vi "motor run.vi"(8 "error in (no error)":errorcluster, 9 "reset":bool, 10 "speed":dbl, 11 "motor in":refnum<class "motor.lvclass">) -> (0 "error out":errorcluster, 3 "motor out":refnum<class "motor.lvclass">)   [LabVIEW 2019, in "my FPGA lib.lvlib" / "motor.lvclass"]
uses:
  motor.lvclass
  motor.lvclass/motor.ctl
  control/PID control.ctl
panel:
  out "motor encoder(degrees)":dbl
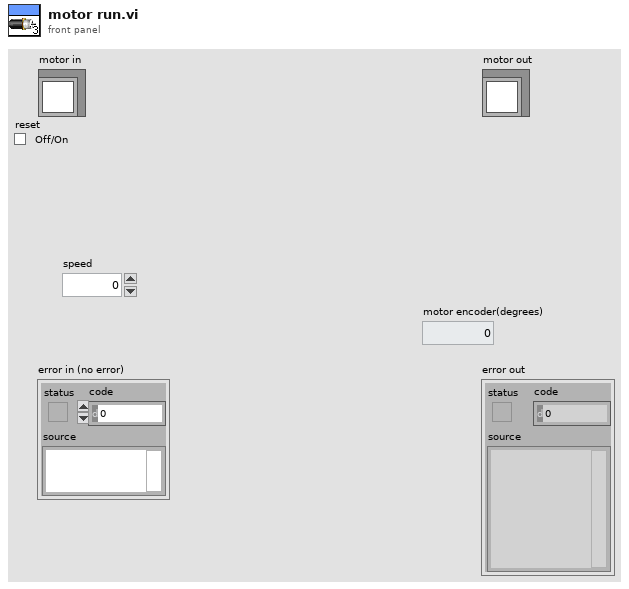
[diagram p1: front panel]
types:
  T1 = typedef "my FPGA lib.lvlib/motor.lvclass/PID control.ctl" = cluster{"setpoint":dbl, "processer":dbl, "last output":dbl}
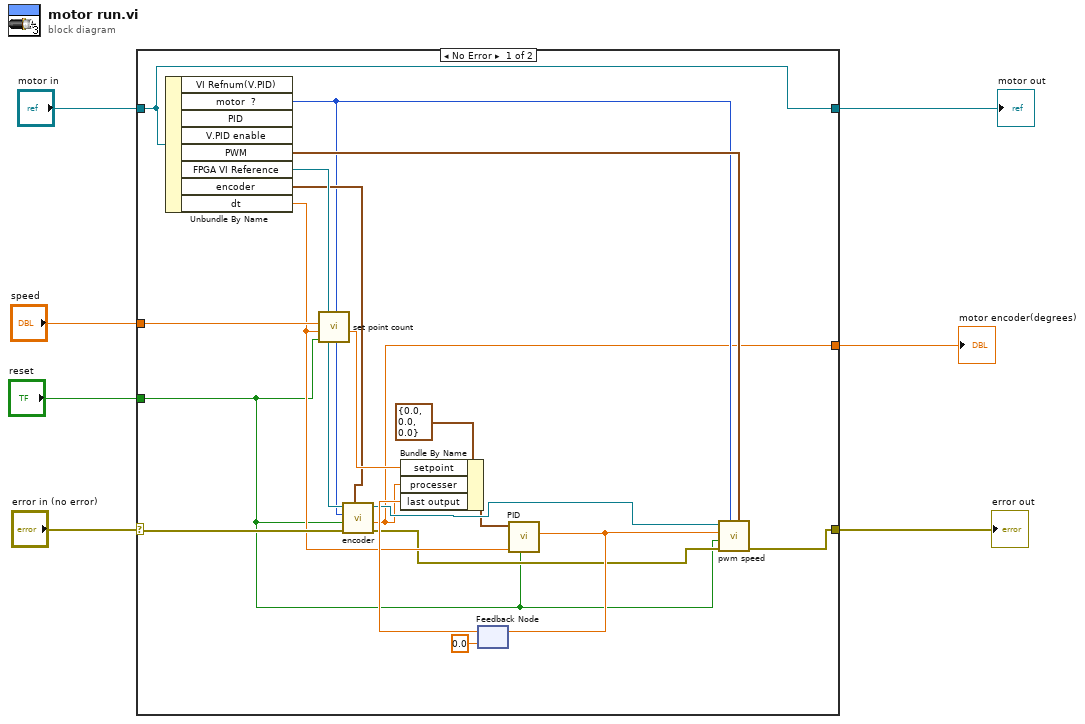
[diagram p0: block diagram]
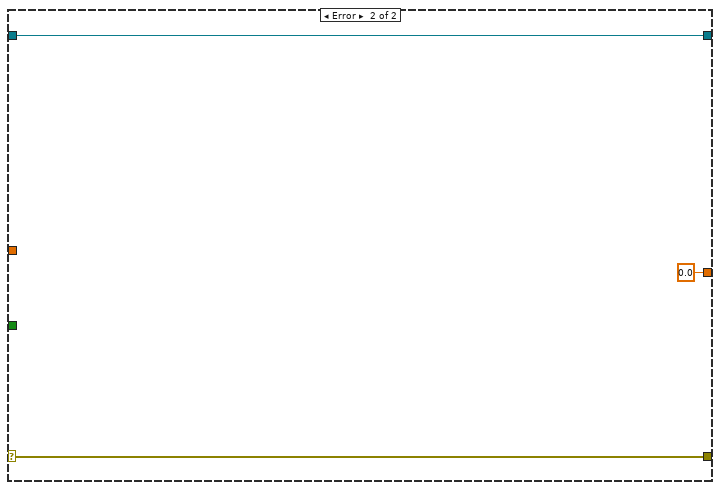
[diagram p2: hidden frame]
diagram:
  n1 = case shown="No Error" "error in (no error)" {
    selector: "error in (no error)" -> [w26 w29]
    tunnel: [w13 w29] -> w6
    tunnel: [w17 w28] -> w4
    tunnel: "motor in" -> [w17 w28]
    tunnel: "reset" -> [w8 _]
    tunnel: "speed" -> [w24 _]
    tunnel: [w12 0.0 ("Motor.encoder")] -> w1
    frame No Error {
      n2 = Unbundle By Name(w17) -> ("motor  ?"=w14:enum16{"M1", "M2", "M3", "M4"}, "PWM"=w15:cluster{"divider":i32, "period":i32}, "FPGA VI Reference"=w25:refnum<k20>, "encoder"=w21:cluster{"encoder PPR":dbl, "gear ratio":dbl}, "dt"=w18:dbl)  [unwired: 3 out]
      n3 = call "set point count.vi"("reset"=w8, "dt(s)"=w18, "speed"=w24) -> ("setpoint"=w22:dbl)  [unwired: 8 in]
      n4 = call "encoder.vi"("encoder"=w21, "error in"=w26, "encoder reset"=w8, "motor  ?"=w14, "FPGA VI Reference"=w25) -> ("error out"=w9:errorcluster, "Motor.encoder"=w12:dbl, "FPGA VI Reference Out"=w16:refnum<k20>)  [unwired: 4 in]
      n5 = feedback #1(0.0 ("output")) -> (w20:dbl)
      n6 = Bundle By Name(cluster=T1 {"setpoint"=0.0, "processer"=0.0, "last output"=0.0} ("control"), "setpoint"=w22, "processer"=w12, "last output"=w20) -> (w10:T1)
      n7 = call "PID.vi"("reinitialize? (F)"=w8, "dt (s)"=w18, "control"=w10) -> ("output"=w11:dbl)  [unwired: 8 in]
      n8 = feedback-in #1(w11) -> ()
      n9 = call "pwm speed.vi"("PWM"=w15, "motor  ?"=w14, "error in"=w9, "brake"=w8, "speed"=w11, "FPGA VI Reference"=w16) -> ("error out"=w13:errorcluster)  [unwired: 4 in, 1 out]
    }
    frame Error {
    }
  }
  "error out" <- w6
  "motor out" <- w4
  "motor encoder(degrees)" <- w1
